vi "Configure Adjacent Channel Power (Offset Setup).vi"(0 "VISA resource name":refnum<visa-resource-name>, 1 "ACP Offset Channel (0:Channel 1)":u16(ring) items=["Channel 1", "Channel 2", "Channel 3"], 2 "ACP Offset State(1:On)":i32(ring)=1 items=["Off", "On"], 3 "ACP Offset Frequency (5000000Hz)":dbl=5000000.0 min=-1000000000.0 max=1000000000.0, 5 "ACP Offset Mode (0:Normal)":i32(ring) items=["Normal", "Advanced"], 7 "ACP Frequency (5000000Hz)":dbl=5000000.0 min=-1000000000.0 max=1000000000.0, 9 "ACP Bandwidth (3840000Hz)":dbl=3840000.0 min=1.0 max=1000000000.0, 11 "error in (no error)":errorcluster) -> (4 "VISA resource name out":refnum<visa-resource-name>, 15 "error out":errorcluster)   [LabVIEW 2020, in "Anritsu Signal Analyzer Series.lvlib"]
doc: "Configures the offset for ACP measurement of the spectrum analyzer."
uses:
  Anritsu Signal Analyzer Series.lvlib
panel:
  # "Hz"
  # "Hz"
  # "Hz"
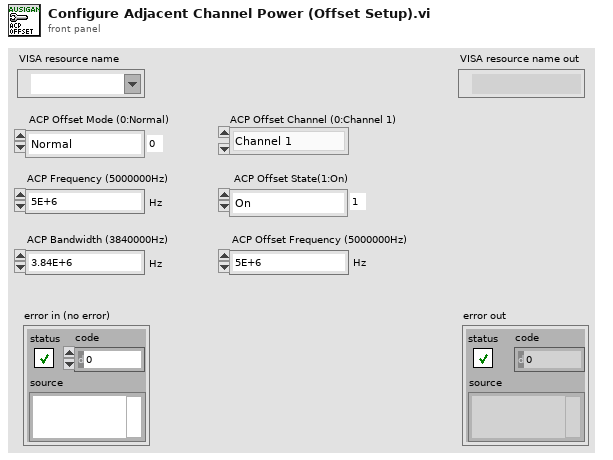
[diagram p1: front panel]
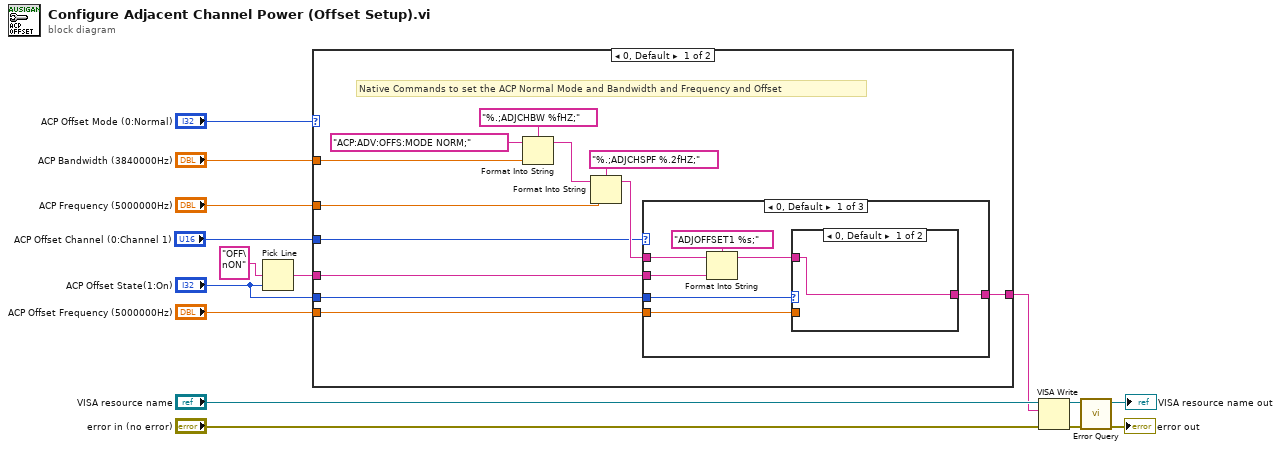
[diagram p0: block diagram]
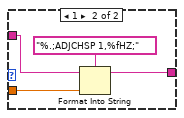
[diagram p2: hidden frame]
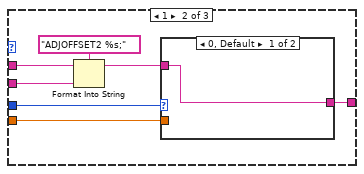
[diagram p3: hidden frame]
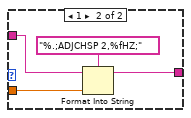
[diagram p4: hidden frame]
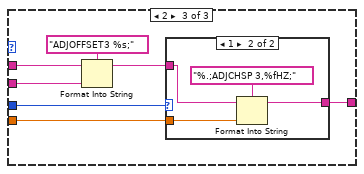
[diagram p5: hidden frame]
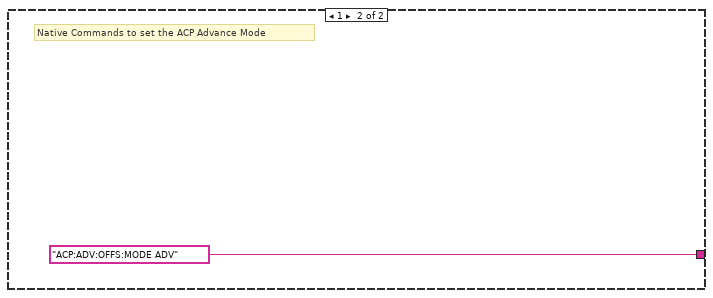
[diagram p7: hidden frame]
diagram:
  n1 = Pick Line(multi-line string="OFF\nON" ("複数行文字列"), line index="ACP Offset State(1:On)") -> (output string=w3:string)  [unwired: 1 in]
  n2 = case shown="0, Default" "ACP Offset Mode (0:Normal)" {
    tunnel: "ACP Bandwidth (3840000Hz)" -> [w26 _]
    tunnel: w3 -> [w22 _]
    tunnel: "ACP Offset Frequency (5000000Hz)" -> [w21 _]
    tunnel: [w17 "ACP:ADV:OFFS:MODE ADV" ("_CommandSet")] -> w5
    tunnel: "ACP Frequency (5000000Hz)" -> [w19 _]
    tunnel: "ACP Offset Channel (0:Channel 1)" -> [w18 _]
    tunnel: "ACP Offset State(1:On)" -> [w16 _]
    frame 0, Default {
      # "Native Commands to set the ACP Normal Mode and Bandwidth and Frequency and Offset"
      n3 = Format Into String(format string="%.;ADJCHBW %fHZ;" ("Format String"), initial string="ACP:ADV:OFFS:MODE NORM;" ("_CommandSet"), w26) -> (resulting string=w24:string)  [unwired: 1 in, 1 out]
      n4 = Format Into String(format string="%.;ADJCHSPF %.2fHZ;" ("Format String"), initial string=w24, w19) -> (resulting string=w23:string)  [unwired: 1 in, 1 out]
      n5 = case shown="0, Default" w18 {
        tunnel: w23 -> [w34 w46 w58]
        tunnel: w22 -> [w32 w44 w56]
        tunnel: w21 -> [w30 w42 w54]
        tunnel: [w29 w41 w53] -> w17
        tunnel: w16 -> [w28 w40 w52]
        frame 0, Default {
          n6 = Format Into String(format string="ADJOFFSET1 %s;" ("_CommandSet"), initial string=w34, w32) -> (resulting string=w31:string)  [unwired: 1 in, 1 out]
          n7 = case shown="0, Default" w28 {
            tunnel: w31 -> [w35 w39]
            tunnel: w30 -> [_ w37]
            tunnel: [w35 w36] -> w29
            frame 0, Default {
            }
            frame 1 {
              n8 = Format Into String(format string="%.;ADJCHSP 1,%fHZ;" ("Format String"), initial string=w39, w37) -> (resulting string=w36:string)  [unwired: 1 in, 1 out]
            }
          }
        }
        frame 1 {
          n9 = Format Into String(format string="ADJOFFSET2 %s;" ("_CommandSet"), initial string=w46, w44) -> (resulting string=w43:string)  [unwired: 1 in, 1 out]
          n10 = case shown="0, Default" w40 {
            tunnel: w43 -> [w47 w51]
            tunnel: w42 -> [_ w49]
            tunnel: [w47 w48] -> w41
            frame 0, Default {
            }
            frame 1 {
              n11 = Format Into String(format string="%.;ADJCHSP 2,%fHZ;" ("Format String"), initial string=w51, w49) -> (resulting string=w48:string)  [unwired: 1 in, 1 out]
            }
          }
        }
        frame 2 {
          n12 = Format Into String(format string="ADJOFFSET3 %s;" ("_CommandSet"), initial string=w58, w56) -> (resulting string=w55:string)  [unwired: 1 in, 1 out]
          n13 = case shown="1" w52 {
            tunnel: w55 -> [w59 w63]
            tunnel: w54 -> [_ w61]
            tunnel: [w59 w60] -> w53
            frame 0, Default {
            }
            frame 1 {
              n14 = Format Into String(format string="%.;ADJCHSP 3,%fHZ;" ("Format String"), initial string=w63, w61) -> (resulting string=w60:string)  [unwired: 1 in, 1 out]
            }
          }
        }
      }
    }
    frame 1 {
      # "Native Commands to set the ACP Advance Mode"
    }
  }
  n15 = VISA Write(VISA resource name="VISA resource name", write buffer=w5, error in (no error)="error in (no error)") -> (VISA resource name out=w7:refnum<visa-resource-name>, error out=w6:errorcluster)  [unwired: 1 out]
  n16 = call "Error Query.vi"("error in (no error)"=w6, "VISA resource name"=w7) -> ("error out"=→"error out":errorcluster, "VISA resource name out"=→"VISA resource name out":refnum<visa-resource-name>)  [unwired: 6 in, 2 out]
